vi "preprocess.vi"(8 "error in (no error)":errorcluster, 10 "image file path":path, 11 "SegmenterDL100224ThreeD in":refnum<class "SegmenterDL100224ThreeD.lvclass">) -> (0 "error out":errorcluster, 2 "preprocessed file path":path, 3 "SegmenterDL100224ThreeD out":refnum<class "SegmenterDL100224ThreeD.lvclass">)   [LabVIEW 2010, in "SegmenterDL100224ThreeD.lvclass"]
uses:
  SegmenterDL100224ThreeD.lvclass
  SegmenterDL100224ThreeD.lvclass/SegmenterDL100224ThreeD.ctl
panel:
  out "console input":string
  out "console output":string
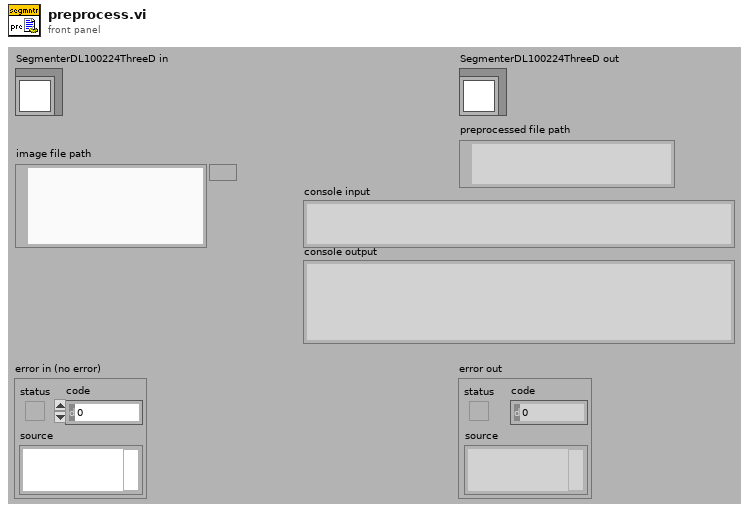
[diagram p1: front panel]
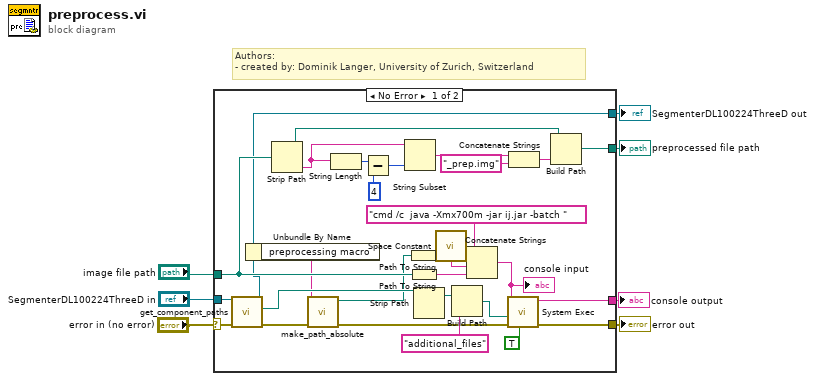
[diagram p0: block diagram]
diagram:
  # "Authors: \n- created by: Dominik Langer, University of Zurich, Switzerland"
  n1 = case shown="No Error" "error in (no error)" {
    selector: "error in (no error)" -> [w20 w38]
    tunnel: [w30 w38] -> w6
    tunnel: [w16 w37] -> w4
    tunnel: "SegmenterDL100224ThreeD in" -> [w31 w37]
    tunnel: "image file path" -> [w18 _]
    tunnel: [w29 _] -> w2
    tunnel: [w22 _] -> w1
    frame No Error {
      n2 = call-dynamic "get_component_paths.vi"("error in (no error)"=w20, "GenericComponent in"=w31) -> ("error out"=w14:errorcluster, "specific component directory"=w15:path, "GenericComponent out"=w16:refnum<class "SegmenterDL100224ThreeD.lvclass">)  [unwired: 4 in, 3 out]
      n3 = Unbundle By Name(w16) -> ("preprocessing macro"=w12:string)
      n4 = Strip Path(path=w18) -> (stripped path=w21:path, name=w17:string)
      n5 = call "make_path_absolute.vi"("error in (no error)"=w14, "relative path"=w12) -> ("error out"=w13:errorcluster, "absolute path"=w10:path)  [unwired: 8 in]
      n6 = String Length(string=w17) -> (length=w23:i32)
      n7 = Subtract(x=w23, y=4) -> (x-y=w25:i32)
      n8 = String Subset(string=w17, length (rest)=w25) -> (substring=w28:string)  [unwired: 1 in]
      n9 = Path To String(path=w10) -> (string=w9:string)
      n10 = Path To String(path=w18) -> (string=w32:string)
      n11 = Strip Path(path=w15) -> (stripped path=w35:path)  [unwired: 1 out]
      n12 = call <vilib>:"Space Constant.vi"() -> ("String"=w8:string)
      n13 = Build Path(base path=w35, name or relative path="additional_files") -> (appended path=w19:path)
      n14 = Concatenate Strings("cmd /c  java -Xmx700m -jar ij.jar -batch ", w9, w8, w32) -> (w33:string)
      "console input" <- w33
      n15 = call <vilib>:"System Exec.vi"("run minimized? (F)"=TRUE, "error in (no error)"=w13, "working directory"=w19, "command line"=w33) -> ("error out"=w30:errorcluster, "standard output"=w29:string)  [unwired: 4 in, 2 out]
      n16 = Concatenate Strings(w28, "_prep.img" ("string")) -> (w27:string)
      n17 = Build Path(base path=w21, name or relative path=w27) -> (appended path=w22:path)
    }
    frame Error {
    }
  }
  "error out" <- w6
  "SegmenterDL100224ThreeD out" <- w4
  "preprocessed file path" <- w1
  "console output" <- w2
